vi "atividade 2 Condicional Enquanto.vi"() -> ()   [LabVIEW 2024]
uses:
  Control 2.ctl
panel:
  in  "Boolean 2":bool
  in  "Celsius":T1 scale=0.0..100.0
  in  "stop 3":bool
  out "Contador":i32
  out "Fahr":dbl(slide) scale=0.0..100.0
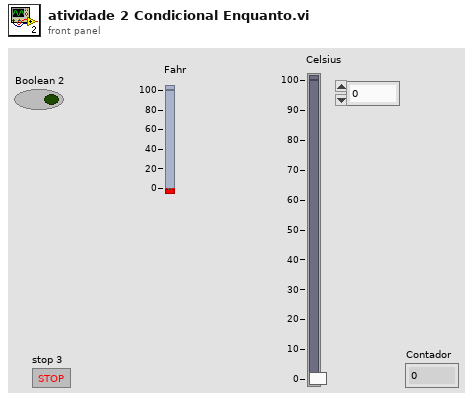
[diagram p1: front panel]
types:
  T1 = typedef "Control 2.ctl" = dbl
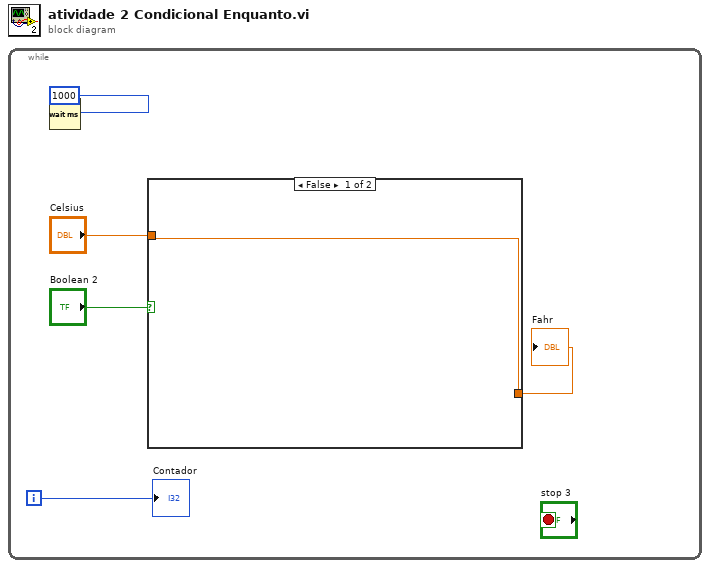
[diagram p0: block diagram]
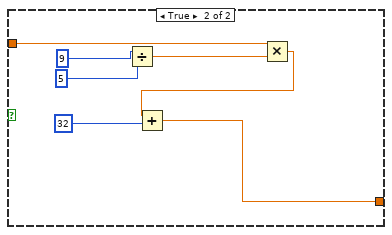
[diagram p2: hidden frame]
diagram:
  n1 = while {
    i -> [w5]
    stop <- "stop 3" stop-if-true
    n2 = Wait (ms)(milliseconds to wait=u32 1000) -> ()  [unwired: 1 out]
    n3 = case shown="False" "Boolean 2" {
      tunnel: "Celsius" -> [w7 w11]
      tunnel: [w7 w10] -> w2
      frame False {
      }
      frame True {
        n4 = Divide(x=9, y=5) -> (x/y=w9:dbl)
        n5 = Multiply(x=w11, y=w9) -> (x*y=w13:T1)
        n6 = Add(x=w13, y=32) -> (x+y=w10:T1)
      }
    }
    "Fahr" <- w2
    "Contador" <- w5
  }
